vi "Rename_setWaveformEvents.vi"(1 "setWaveform":refnum<user-event>[](array[refnum])) -> (0 "setWaveform":refnum<user-event>[](array[refnum]))   [LabVIEW 2020, in "DAQ_Manager.lvclass"]
uses:
  DAQ_Manager.lvclass
  DAQ/Typedefs/PublicEvents--DAQ.Read.ctl
  DAQ/DAQ.lvclass
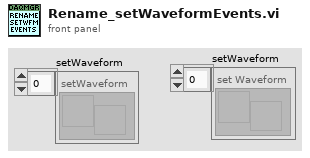
[diagram p1: front panel]
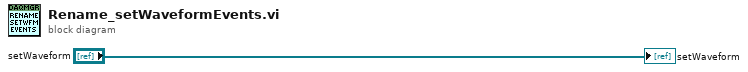
[diagram p0: block diagram]
diagram:
  "setWaveform" <- "setWaveform"
